vi "sub_frame_bu.vi"(8 "felharmonikus N":i32=2, 9 "SNR window width [Hz]":dbl=0.4 format="%#_13g", 11 "path to binary file":path) -> (3 "output cluster":T1)   [LabVIEW 2017]
uses:
  <vilib>/Utility/file.llb/Read Delimited Spreadsheet (string).vi
  <vilib>/regexp/Match Regular Expression.xnode
panel:
  out "header":T2
  out "impulse szum/time (bigger better)":cluster{"X":dbl, "Y":dbl}[](graph)
  out "X SNR 3 (bigger better)":cluster{"X":dbl, "Y":dbl}[](graph)
  out "X SNR 4":cluster{"X":dbl, "Y":dbl}[](graph)
  out "X SNR":cluster{"X":dbl, "Y":dbl}[](graph)
  out "impulse mean (?)":cluster{"X":dbl, "Y":dbl}[](graph)
  out "impulse sd (?)":cluster{"X":dbl, "Y":dbl}[](graph)
  out "impulse szum (?)":cluster{"X":dbl, "Y":dbl}[](graph)
  out "enable":bool
  out "end":timestamp
  out "start":timestamp
  out "state":string
  out "saved":string
  out "all rows":string[][](array[string])
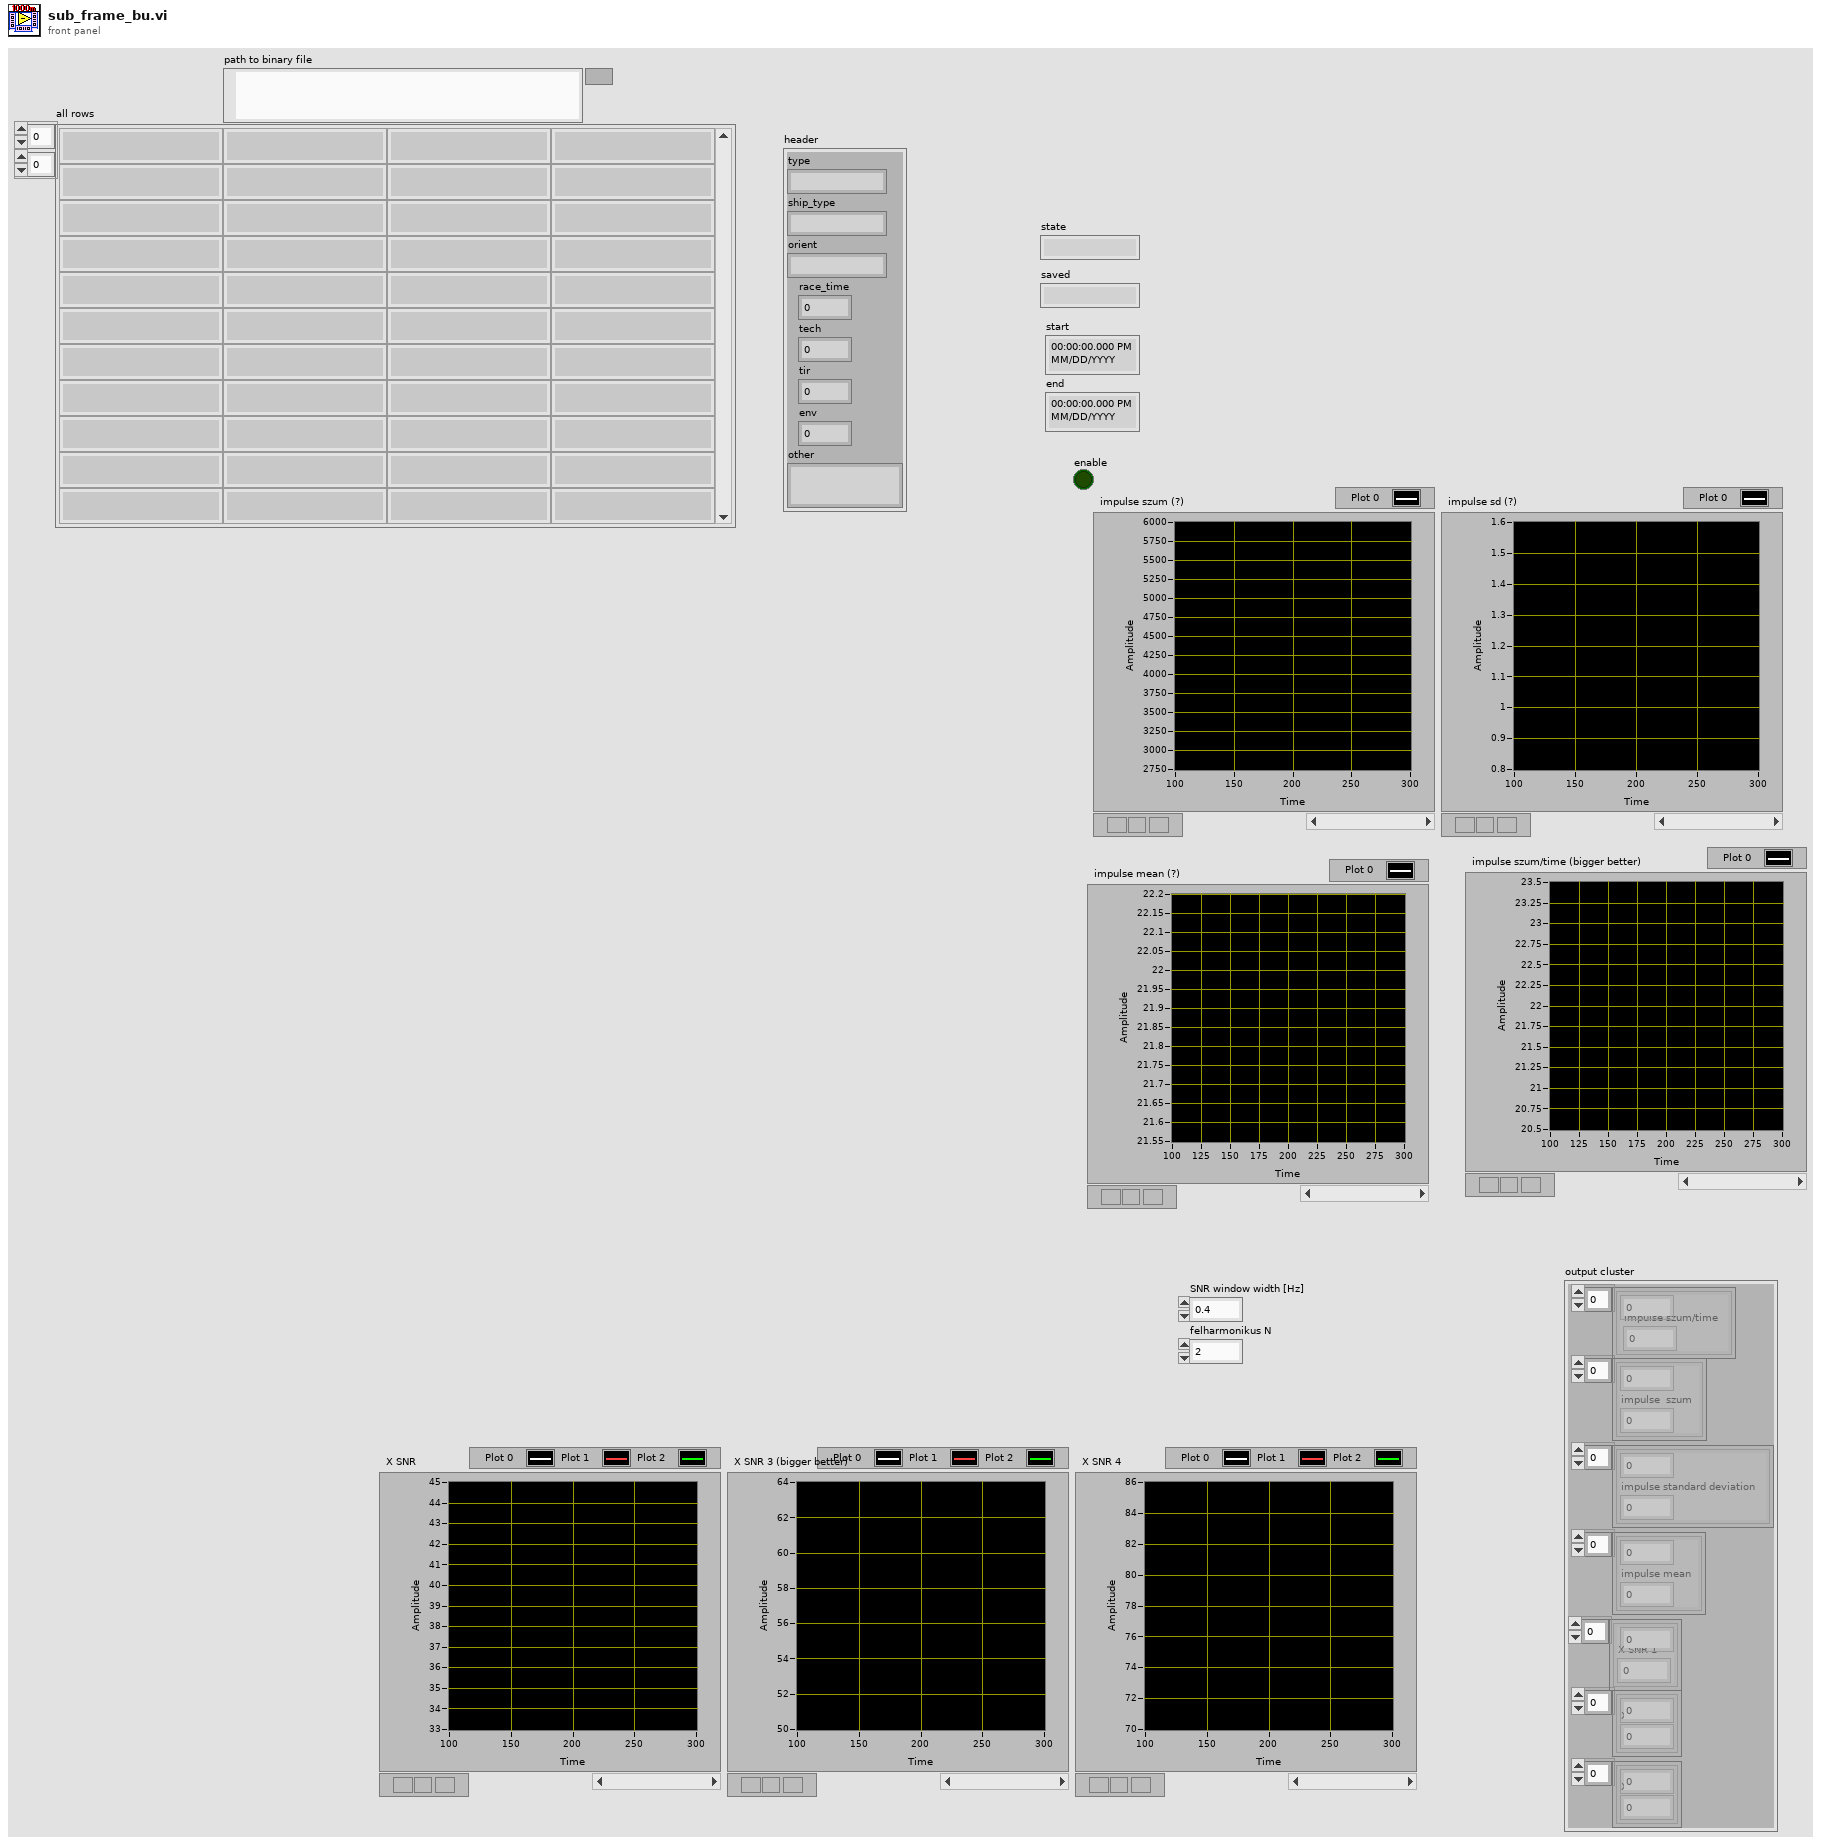
[diagram p1: front panel]
types:
  T1 = cluster{cluster{dbl, "impulse szum/time":dbl}[], cluster{dbl, "impulse  szum":dbl}[], cluster{dbl, "impulse standard deviation":dbl}[], cluster{dbl, "impulse mean":dbl}[], cluster{dbl, "X SNR 1":dbl}[], cluster{dbl, "X SNR 2":dbl}[], cluster{dbl, "X SNR 3":dbl}[]}
  T2 = cluster{"type":string, "ship_type":string, "orient":string, "race_time":dbl, "tech":dbl, "tir":dbl, "env":dbl, "other":string}
  T3 = cluster{cluster{dbl, "impulse szum/time":dbl}[], cluster{dbl, "impulse  szum":dbl}[], cluster{dbl, "impulse standard deviation":dbl}[], cluster{dbl, "impulse mean":dbl}[], cluster{dbl, dbl}[], cluster{dbl, dbl}[], cluster{dbl, dbl}[]}
  T4 = cluster{"path to binary file":path, "Start Cursor":timestamp, "Sec":dbl, "crossing level":dbl, "threshold":dbl, "avg window size":i32, "peak detect width":i32, "invert":bool, "SNR window width [Hz]":dbl, "felharmonikus N":i32, "End cursor":timestamp}
  T5 = cluster{"Átlag Csapásszám [stroke/m]":dbl, "mean of peaks":dbl, "impulse standard deviation":dbl, "impulse  szum":dbl, "standard deviation of peaks":dbl, "impulse mean":dbl, "X axis SNR mean":dbl, "X axis SNR standard deviation":dbl, "Y axis SNR standard deviation":dbl, "Y axis SNR mean":dbl, "resultant SNR standard deviation":dbl, "resultant SNR mean":dbl, "Z axis SNR standard deviation":dbl, "Z axis SNR mean":dbl, "impulse szum/mean":dbl}
  T6 = cluster{"Átlag Csapásszám [stroke/m]":dbl, "mean of peaks":dbl, "impulse standard deviation":dbl, "impulse  szum":dbl, "standard deviation of peaks":dbl, "impulse mean":dbl, "X axis SNR mean":dbl, "X axis SNR standard deviation":dbl, "Y axis SNR standard deviation":dbl, "Y axis SNR mean":dbl, "resultant SNR standard deviation":dbl, "resultant SNR mean":dbl, "Z axis SNR standard deviation":dbl, "Z axis SNR mean":dbl, "impulse szum/mean":dbl}[]
  T7 = cluster{cluster{dbl, dbl}[], cluster{dbl, "impulse  szum":dbl}[], cluster{dbl, "impulse standard deviation":dbl}[], cluster{dbl, "impulse mean":dbl}[], cluster{dbl, dbl}[], cluster{dbl, dbl}[], cluster{dbl, dbl}[]}
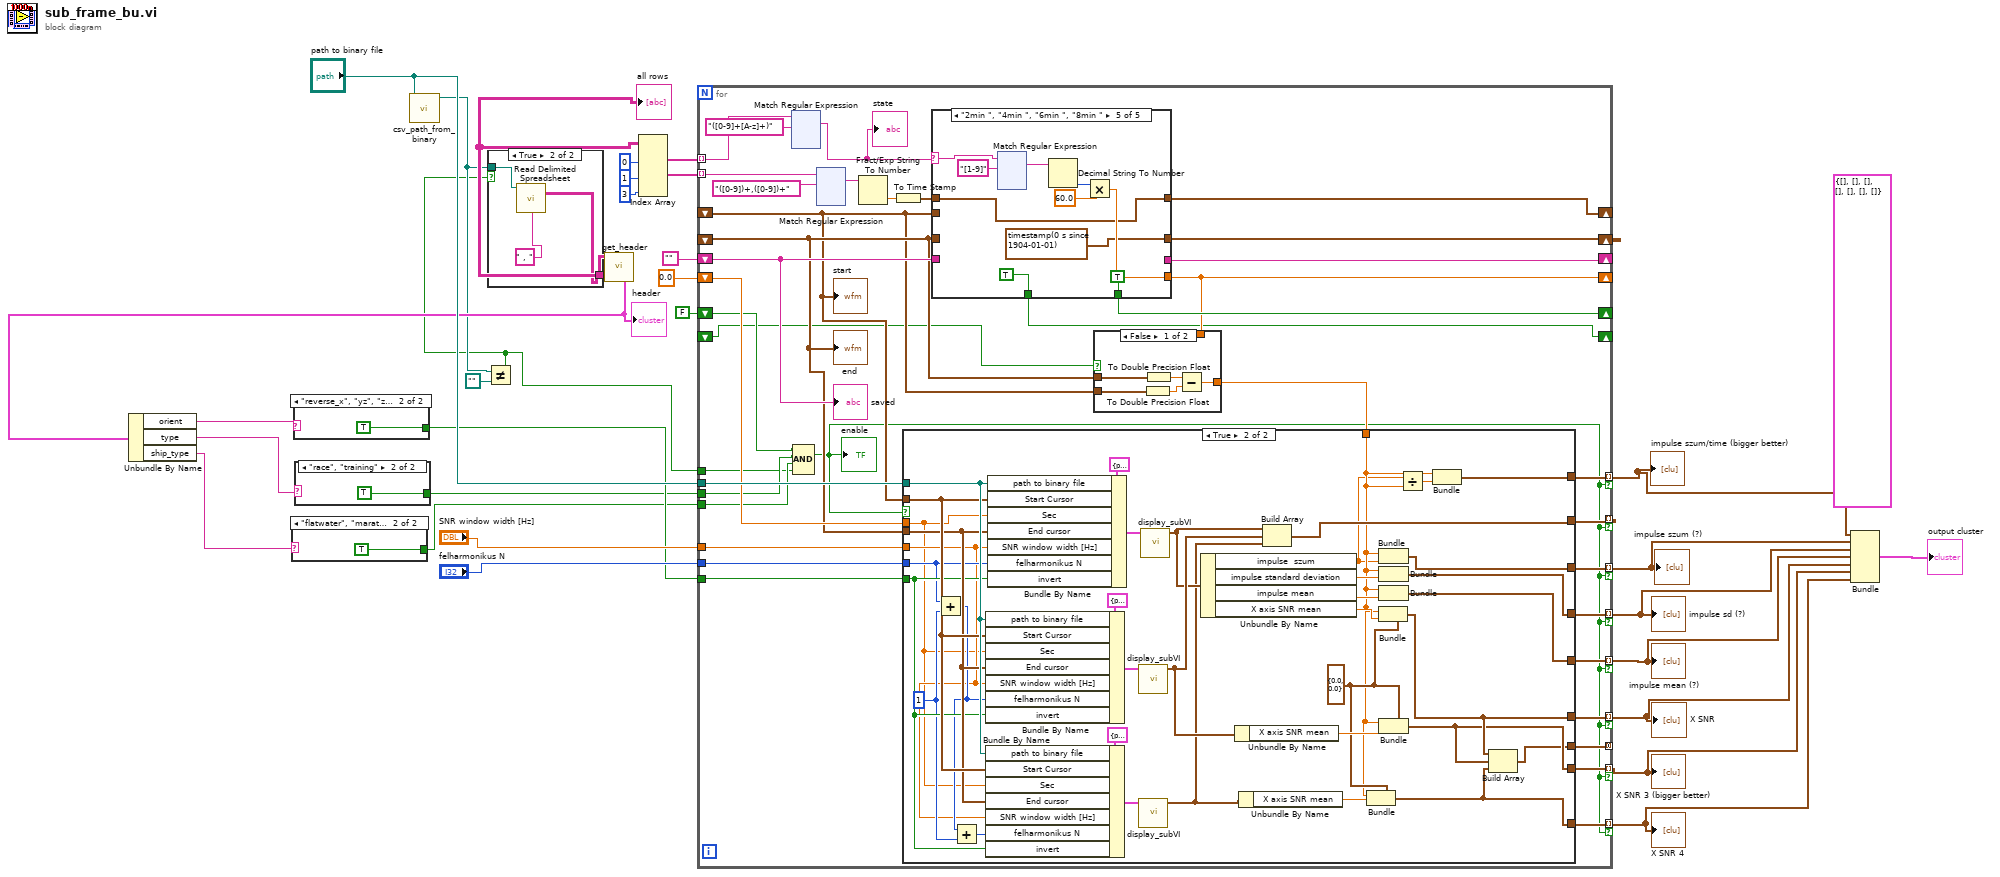
[diagram p0: block diagram]
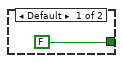
[diagram p3: hidden frame]
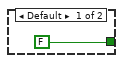
[diagram p4: hidden frame]
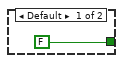
[diagram p5: hidden frame]
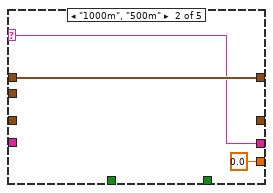
[diagram p9: hidden frame]
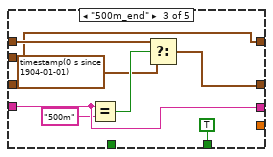
[diagram p10: hidden frame]
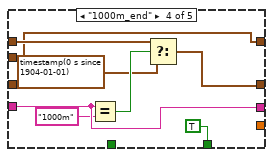
[diagram p11: hidden frame]
diagram:
  (unwired) T3 {[], [], [], [], [], [], []} ("output cluster")
  n1 = call "csv_path_from_binary.vi"("path to binary file"="path to binary file") -> ("path to spec. ext."=w3:path)  [unwired: 10 in]
  n2 = Not Equal?(x=w3, y=path "") -> (x != y?=w2:bool)
  n3 = case shown="True" w2 {
    tunnel: [_ w32] -> w4
    tunnel: w3 -> [_ w31]
    frame False {
    }
    frame True {
      n4 = call-poly <vilib>:"Read Delimited Spreadsheet.vi"("file path (dialog if empty)"=w31, "delimiter (\\t)"=" , " ("delimiter (\\t)")) -> ("all rows"=w32:string[][])  [unwired: 8 in, 5 out]
    }
  }
  "all rows" <- w4
  n5 = call "get_header.vi"("all rows"=w4) -> ("header"=w20:T2)  [unwired: 10 in]
  "header" <- w20
  n6 = Unbundle By Name(w20) -> ("orient"=w19:string, "type"=w9:string, "ship_type"=w7:string)
  n7 = case shown="\"flatwater\", \"marathon\"" w7 {
    tunnel: [FALSE TRUE] -> w6
    frame Default {
    }
    frame "flatwater", "marathon" {
    }
  }
  n8 = case shown="\"reverse_x\", \"yz\", \"z\"" w19 {
    tunnel: [FALSE TRUE] -> w18
    frame Default {
    }
    frame "reverse_x", "yz", "z" {
    }
  }
  n9 = case shown="\"race\", \"training\"" w9 {
    tunnel: [FALSE TRUE] -> w8
    frame Default {
    }
    frame "race", "training" {
    }
  }
  n10 = Index Array(array=w4, index (col) #1=0 ("disabled index (col)"), index (col) #2=1 ("index (col)"), index (col) #3=3 ("index (row)")) -> (element #1=w29:string[], element #2=w30:string[])  [unwired: 3 in, 1 out]
  n11 = for {
    tunnel: w30 -> [w74] mode=indexing
    tunnel: w29 -> [w69] mode=indexing
    shift-right: [w72] -> _
    shift-left: _ -> [w58]
    shift-right: [w71] -> _
    shift-left: _ -> [w59]
    shift-right: [w70] -> _
    shift-left: "" -> [w66]
    shift-right: [w42] -> _
    shift-left: 0.0 ("Sec") -> [w63]
    shift-right: [w65] -> _
    shift-left: FALSE -> [w46]
    tunnel: "path to binary file" -> [w64]
    tunnel: "SNR window width [Hz]" -> [w62]
    tunnel: "felharmonikus N" -> [w61]
    tunnel: w18 -> [w60]
    tunnel: [w56] -> _ mode=indexing if=w47
    tunnel: [w55] -> w16 mode=indexing if=w47
    tunnel: [w54] -> w15 mode=indexing if=w47
    tunnel: [w53] -> w14 mode=indexing if=w47
    tunnel: [w52] -> w13 mode=indexing if=w47
    tunnel: [w51] -> w12 mode=indexing if=w47
    tunnel: [w50] -> w11 mode=indexing if=w47
    tunnel: [w49] -> _ mode=concatenating
    tunnel: [w48] -> w17 mode=indexing if=w47
    tunnel: w8 -> [w45]
    tunnel: w6 -> [w44]
    tunnel: w2 -> [w43]
    shift-right: [w41] -> _
    shift-left: _ -> [w40]
    n12 = xnode "Match Regular Expression"("input string"=w69, "regular expression"="([0-9]+[A-z]+)") -> ("whole match"=w67:string)  [unwired: 4 in, 4 out]
    "state" <- w67
    n13 = Compound Arithmetic op=AND(w46, w45, w44, w43) -> (w47:bool)
    "enable" <- w47
    n14 = xnode "Match Regular Expression"("input string"=w74, "regular expression"="([0-9])+,([0-9])+") -> ("whole match"=w76:string)  [unwired: 4 in, 4 out]
    n15 = Fract/Exp String To Number(string=w76) -> (number=w75:dbl)  [unwired: 3 in, 1 out]
    n16 = To Time Stamp(1:w75) -> (0:w73:timestamp)
    n17 = case shown="\"2min \", \"4min \", \"6min \", \"8min \"" w67 {
      selector: w67 -> [_ w239 _ _ w265]
      tunnel: [w235 w240 w242 w250 w260] -> w72
      tunnel: w73 -> [_ w240 w247 w255 w260]
      tunnel: [w236 _ w246 w254 timestamp(0 s since 1904-01-01) ("f")] -> w71
      tunnel: [w237 w239 w245 w253 _] -> w70
      tunnel: w66 -> [w237 _ w245 w253 _]
      tunnel: [_ 0.0 _ _ w261] -> w42
      tunnel: w59 -> [w236 _ _ _ _]
      tunnel: w58 -> [w235 _ w242 w250 _]
      tunnel: [_ _ TRUE TRUE TRUE] -> w65
      tunnel: [_ _ _ _ TRUE] -> w41
      frame Default {
      }
      frame "1000m", "500m" {
      }
      frame "500m_end" {
        n18 = Equal?(x=w245, y="500m") -> (x = y?=w248:bool)
        n19 = Select(t=w247, s=w248, f=timestamp(0 s since 1904-01-01)) -> (s? t:f=w246:timestamp)
      }
      frame "1000m_end" {
        n20 = Equal?(x=w253, y="1000m") -> (x = y?=w256:bool)
        n21 = Select(t=w255, s=w256, f=timestamp(0 s since 1904-01-01)) -> (s? t:f=w254:timestamp)
      }
      frame "2min ", "4min ", "6min ", "8min " {
        n22 = xnode "Match Regular Expression"("input string"=w265, "regular expression"="[1-9]") -> ("whole match"=w264:string)  [unwired: 4 in, 4 out]
        n23 = Decimal String To Number(string=w264) -> (number=w262:i32)  [unwired: 2 in, 1 out]
        n24 = Multiply(x=w262, y=60.0) -> (x*y=w261:dbl)
      }
    }
    n25 = case shown="False" w40 {
      tunnel: w59 -> [w82 _]
      tunnel: w58 -> [w81 _]
      tunnel: [w78 w83] -> w57
      tunnel: w42 -> [_ w83]
      frame False {
        n26 = To Double Precision Float(number=w81) -> (double precision float=w79:dbl)
        n27 = To Double Precision Float(number=w82) -> (double precision float=w80:dbl)
        n28 = Subtract(x=w80, y=w79) -> (x-y=w78:dbl)
      }
      frame True {
      }
    }
    n29 = case shown="True" w47 {
      tunnel: w64 -> [_ w114]
      tunnel: w58 -> [_ w113]
      tunnel: w59 -> [_ w112]
      tunnel: w63 -> [_ w105]
      tunnel: w62 -> [_ w106]
      tunnel: w61 -> [_ w110]
      tunnel: w60 -> [_ w111]
      tunnel: w57 -> [_ w85]
      tunnel: [_ w100] -> w56
      tunnel: [_ w99] -> w55
      tunnel: [_ w98] -> w54
      tunnel: [_ w97] -> w53
      tunnel: [_ w92] -> w52
      tunnel: [_ w91] -> w51
      tunnel: [_ w90] -> w50
      tunnel: [_ w89] -> w49
      tunnel: [_ w87] -> w48
      frame False {
      }
      frame True {
        w88 = cluster{dbl, dbl} {0.0, 0.0} ("cluster")
        w107 = 1
        n30 = Add(x=w110, y=w107) -> (x+y=w108:i32)
        n31 = Add(x=w108, y=w107) -> (x+y=w109:i32)
        n32 = Bundle By Name(cluster=T4 {"path to binary file"=path "C:/Users/Lenovo/Desktop/szakdoga/data", "Start Cursor"=timestamp(0 s since 1904-01-01), "Sec"=60.0, "crossing level"=0.0, "threshold"=0.35, "avg window size"=5, "peak detect width"=30, "invert"=FALSE, "SNR window width [Hz]"=0.5, "felharmonikus N"=2, "End cursor"=timestamp(0 s since 1904-01-01)} ("input cluster"), "path to binary file"=w114, "Start Cursor"=w113, "Sec"=w105, "End cursor"=w112, "SNR window width [Hz]"=w106, "felharmonikus N"=w108, "invert"=w111) -> (w117:T4)
        n33 = Bundle By Name(cluster=T4 {"path to binary file"=path "C:/Users/Lenovo/Desktop/szakdoga/data", "Start Cursor"=timestamp(0 s since 1904-01-01), "Sec"=60.0, "crossing level"=0.0, "threshold"=0.35, "avg window size"=5, "peak detect width"=30, "invert"=FALSE, "SNR window width [Hz]"=0.5, "felharmonikus N"=2, "End cursor"=timestamp(0 s since 1904-01-01)} ("input cluster"), "path to binary file"=w114, "Start Cursor"=w113, "Sec"=w105, "End cursor"=w112, "SNR window width [Hz]"=w106, "felharmonikus N"=w109, "invert"=w111) -> (w116:T4)
        n34 = Bundle By Name(cluster=T4 {"path to binary file"=path "C:/Users/Lenovo/Desktop/szakdoga/data", "Start Cursor"=timestamp(0 s since 1904-01-01), "Sec"=60.0, "crossing level"=0.0, "threshold"=0.35, "avg window size"=5, "peak detect width"=30, "invert"=FALSE, "SNR window width [Hz]"=0.5, "felharmonikus N"=2, "End cursor"=timestamp(0 s since 1904-01-01)} ("input cluster"), "path to binary file"=w114, "Start Cursor"=w113, "Sec"=w105, "End cursor"=w112, "SNR window width [Hz]"=w106, "felharmonikus N"=w110, "invert"=w111) -> (w120:T4)
        n35 = call "display_subVI.vi"("input cluster"=w117) -> ("data cluster"=w102:T5)  [unwired: 10 in]
        n36 = call "display_subVI.vi"("input cluster"=w116) -> ("data cluster"=w93:T5)  [unwired: 10 in]
        n37 = call "display_subVI.vi"("input cluster"=w120) -> ("data cluster"=w101:T5)  [unwired: 10 in]
        n38 = Unbundle By Name(w101) -> ("impulse  szum"=w84:dbl, "impulse standard deviation"=w103:dbl, "impulse mean"=w104:dbl, "X axis SNR mean"=w96:dbl)
        n39 = Unbundle By Name(w102) -> ("X axis SNR mean"=w95:dbl)
        n40 = Unbundle By Name(w93) -> ("X axis SNR mean"=w94:dbl)
        n41 = Build Array(w101, w102, w93) -> (w100:T6)
        n42 = Bundle(cluster=w88, w85, w94) -> (w90:cluster{dbl, dbl})
        n43 = Bundle(cluster=w88, w85, w96) -> (w92:cluster{dbl, dbl})
        n44 = Bundle(w85, "impulse  szum"=w84) -> (w99:cluster{dbl, "impulse  szum":dbl})  [unwired: 1 in]
        n45 = Bundle(w85, "impulse standard deviation"=w103) -> (w98:cluster{dbl, "impulse standard deviation":dbl})  [unwired: 1 in]
        n46 = Bundle(w85, "impulse mean"=w104) -> (w97:cluster{dbl, "impulse mean":dbl})  [unwired: 1 in]
        n47 = Bundle(cluster=w88, w85, w95) -> (w91:cluster{dbl, dbl})
        n48 = Divide(x=w84, y=w85) -> (x/y=w86:dbl)
        n49 = Bundle(w85, w86) -> (w87:cluster{dbl, dbl})  [unwired: 1 in]
        n50 = Build Array(w92, w91, w90) -> (w89:cluster{dbl, dbl}[])
      }
    }
    "saved" <- w66
    "start" <- w58
    "end" <- w59
  }
  "impulse szum (?)" <- w16
  "impulse sd (?)" <- w15
  "impulse mean (?)" <- w14
  "X SNR" <- w13
  "X SNR 4" <- w11
  "X SNR 3 (bigger better)" <- w12
  "impulse szum/time (bigger better)" <- w17
  n51 = Bundle(w17, w16, w15, w14, w13, w12, w11) -> (→"output cluster":T7)  [unwired: 1 in]
